vi "Calibrate External Adjust.vi"(8 "error in":errorcluster, 10 "Frac Error":dbl, 11 "Instrument Handle In":i32) -> (0 "error out":errorcluster, 3 "Instrument Handle Out":i32)   [LabVIEW 8.6, in "ZTScopeM.lvlib"]
doc: "Adjust the instrument's external trigger calibration settings. See the instrument calibration manual for more information."
uses:
  ZTScopeM.lvlib
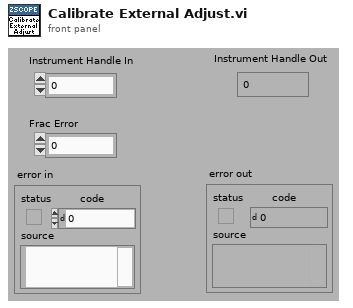
[diagram p1: front panel]
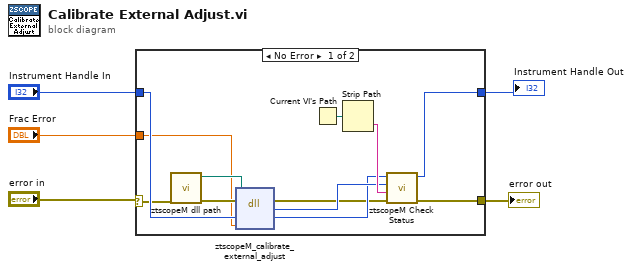
[diagram p0: block diagram]
diagram:
  n1 = case shown="No Error" "error in" {
    selector: "error in" -> [w10 w19]
    tunnel: [w12 w19] -> w2
    tunnel: "Instrument Handle In" -> [w17 w18]
    tunnel: [w11 w18] -> w4
    tunnel: "Frac Error" -> [w6 _]
    frame #0 {
      n2 = call "ztscopeM dll path.vi"("error in (no error)"=w10) -> ("error out"=w8:errorcluster, "<instrument>.dll path"=w9:path)  [unwired: 9 in]
      n3 = dll-call lib="C:/Program Files (x86)/National Instruments/LabVIEW 2013/instr.lib/ztscopem/ztscopeM.dll" fn="ztscopeM_calibrate_external_adjust"(path in=w9, error in=w8, "instrumentHandle"=w17, "Error Correction"=w6) -> (error out=w7:errorcluster, w14:i32, "instrumentHandle"=w13:i32)  [unwired: 2 in, 1 out]
      n4 = Current VI's Path() -> (path=w16:path)
      n5 = Strip Path(path=w16) -> (name=w15:string)  [unwired: 1 out]
      n6 = call "ztscopeM Check Status.vi"("error in"=w7, "name of VI"=w15, "status (return code)"=w14, "instrument handle in"=w13) -> ("error out"=w12:errorcluster, "instrument handle out"=w11:i32)  [unwired: 2 in]
    }
    frame #1 {
    }
  }
  "Instrument Handle Out" <- w4
  "error out" <- w2
